vi "Hello World.vi"() -> ()   [LabVIEW 2018]
panel:
  in  "?":bool
  out "?":string
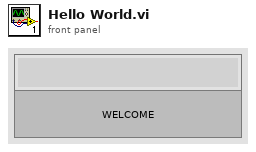
[diagram p1: front panel]
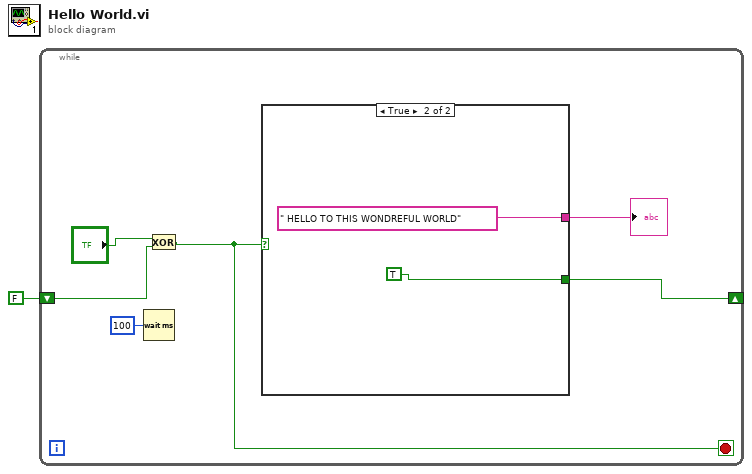
[diagram p0: block diagram]
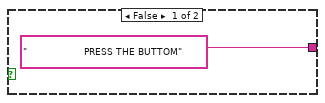
[diagram p2: hidden frame]
diagram:
  n1 = while {
    shift-right: [w5] -> _
    shift-left: FALSE -> [w3]
    stop <- w2 stop-if-true
    n2 = Wait (ms)(milliseconds to wait=u32 100) -> ()  [unwired: 1 out]
    n3 = Exclusive Or(1:w3, 2:"?") -> (0:w2:bool)
    n4 = case shown="True" w2 {
      tunnel: ["                   PRESS THE BUTTOM" " HELLO TO THIS WONDREFUL WORLD"] -> w7
      tunnel: [_ TRUE] -> w5
      frame False {
      }
      frame True {
      }
    }
    "?" <- w7
  }
